vi "Actor Core.vi"(8 "error in":errorcluster, 11 "Multiharp in":refnum<class "Multiharp.lvclass">) -> (0 "error out":errorcluster, 3 "Actor out":refnum<class "Actor.lvclass">)   [LabVIEW 2023, in "Multiharp.lvlib" / "Multiharp.lvclass"]
doc: "(<B>Filename</B>: Actor Framework.lvlib:Actor.lvclass:Actor Core.vi)\n\nReceives messages to the actor, reacts to them, and initiates any error handling that may shut the actor down.\n\nDescendant classes may override this VI to append parallel tasks for the actor to complete while it handles messages. Overrides use the Call Parent Class Method node."
uses:
  Multiharp.lvclass
  C:/Program Files/National Instruments/LabVIEW 2023/vi.lib/ActorFramework/Actor/Actor.lvclass
  <vilib>/ActorFramework/Actor/Actor.lvclass
  MH_ActorCluster.ctl
  Types/MH_DataProcThread_QData.ctl
  Types/MH_DataProcThread_QCmds.ctl
  UIs/SinglePhoton_UI/Libraries/SinglePhotonInterferenceUI/CountsHistos.ctl
  <vilib>/ActorFramework/Message Enqueuer/Message Enqueuer.lvclass
  <vilib>/ActorFramework/Actor/Actor.lvclass/Actor.ctl
  <vilib>/ActorFramework/Message Enqueuer/Message Enqueuer.lvclass/Message Enqueuer.ctl
  Multiharp.lvclass/Multiharp.ctl
  MultiharpComm Messages/MH_MeasurementDone Msg/MH_MeasurementDone Msg.lvclass/MH_MeasurementDone Msg.ctl
  MultiharpComm Messages/MH_DataInQueue Msg/MH_DataInQueue Msg.lvclass/MH_DataInQueue Msg.ctl
  <vilib>/ActorFramework/Message Enqueuer/Init from Existing Queue.vi
  <vilib>/ActorFramework/Message Enqueuer/Enqueue.vi
  Multiharp Messages/StopMeasurement Msg/StopMeasurement Msg.lvclass
  C:/Program Files/National Instruments/LabVIEW 2023/vi.lib/ActorFramework/Message/Message.lvclass
  MultiharpComm Messages/MH_MeasurementDone Msg/MH_MeasurementDone Msg.lvclass
  MultiharpComm Messages/MH_DataInQueue Msg/MH_DataInQueue Msg.lvclass
  <vilib>/ActorFramework/Message Priority Queue/Priority Enqueue.vi
  typedefs/typedefs.lvlib
panel:
  out "UI Enqueuer":refnum<class "Message Enqueuer.lvclass">
  out "Self Enqueuer":refnum<class "Message Enqueuer.lvclass">
  in  "CountsHistos":T1
  in  "CountsHistos":T1
  in  "FIFO Buffer":T2={"Cmd"=enum."Proc", "nActual"=0, "Buffer"=[], "TickCount"=0, "Param"=0, "Max Triggers"=0, "Coincidence Window"=2.0, "Coincidence Delays"=[], "file path"=path ""}
  in  "MH_ActorCluster":T4={"Histo On"=FALSE, "Initialized"=FALSE, "Acquiring"=FALSE, "ActualHistoLe"=0, "Scanning"=TRUE, "nchannels"=0, "file path"=path "", "BufferSize"=[]}
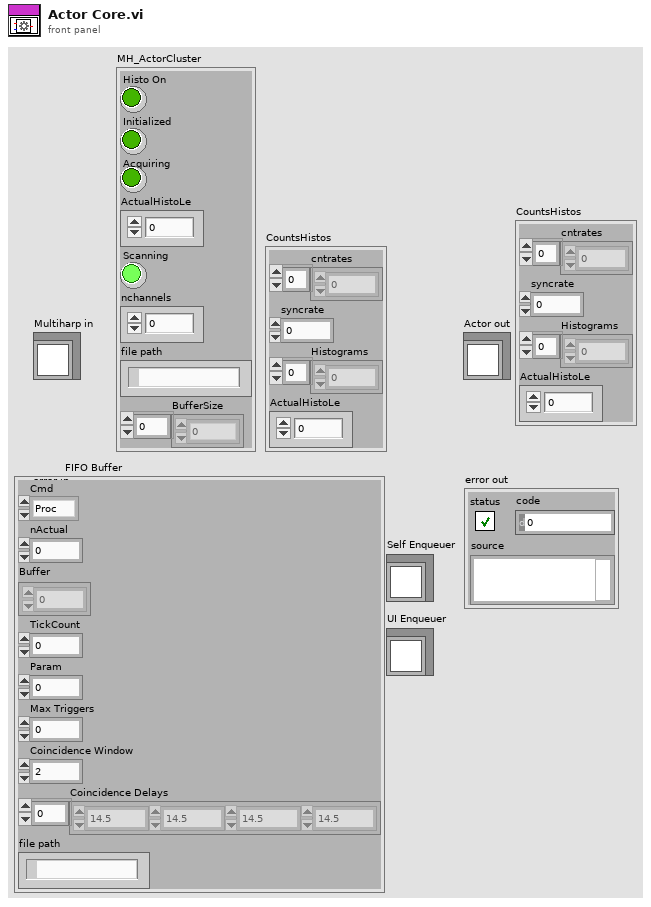
[diagram p1: front panel]
types:
  T1 = typedef "typedefs.lvlib/CountsHistos.ctl" = cluster{"cntrates":i32[], "syncrate":i32, "Histograms":u32[], "ActualHistoLe":i32}
  T2 = typedef "MH_DataProcThread_QData.ctl" = cluster{"Cmd":T3, "nActual":i32, "Buffer":u32[], "TickCount":u32, "Param":i32, "Max Triggers":i32, "Coincidence Window":dbl, "Coincidence Delays":dbl[], "file path":path}
  T3 = typedef "MH_DataProcThread_QCmds.ctl" = enum16{"Exit", "Proc", "Init", "SaveCSV", "SetNumChannels"}
  T4 = typedef "MH_ActorCluster.ctl" = cluster{"Histo On":bool, "Initialized":bool, "Acquiring":bool, "ActualHistoLe":i32, "Scanning":bool, "nchannels":i32, "file path":path, "BufferSize":dbl[]}
  T5 = enum16{"Idle", "Scanning", "Acquiring", "Histogramming", "Counting"}
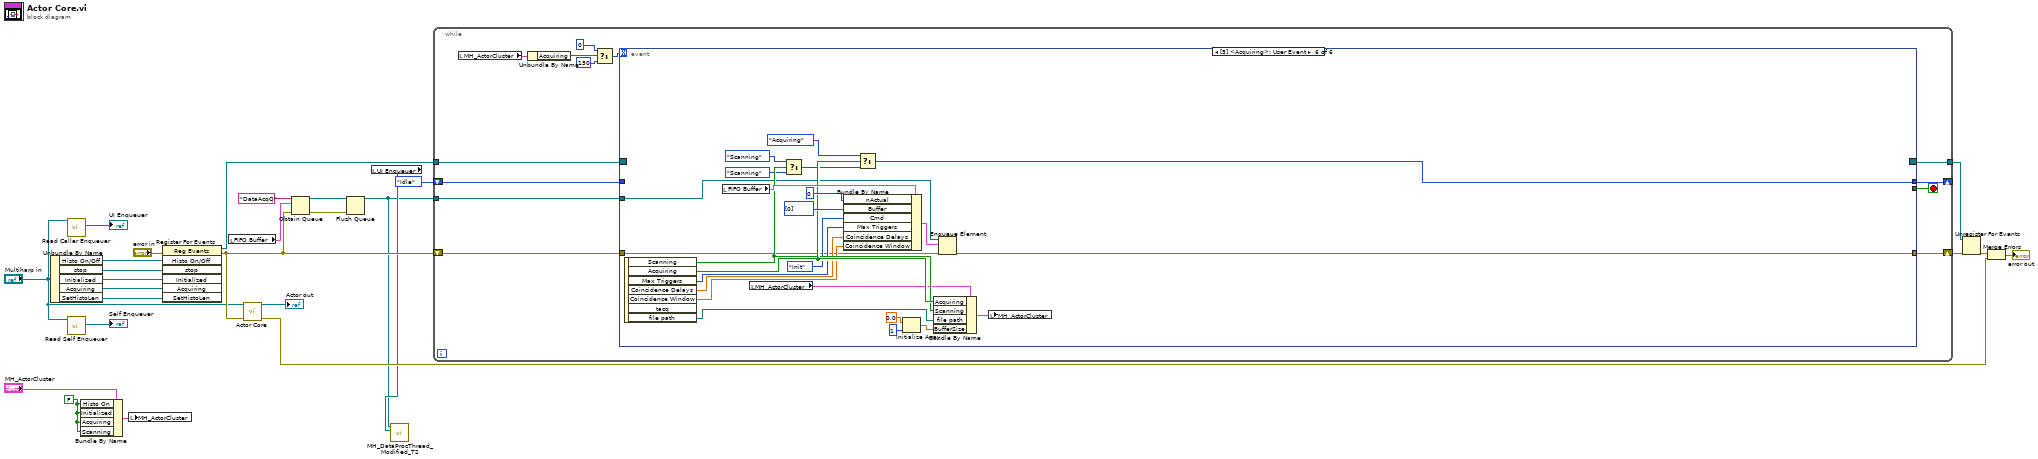
[diagram p0: block diagram]
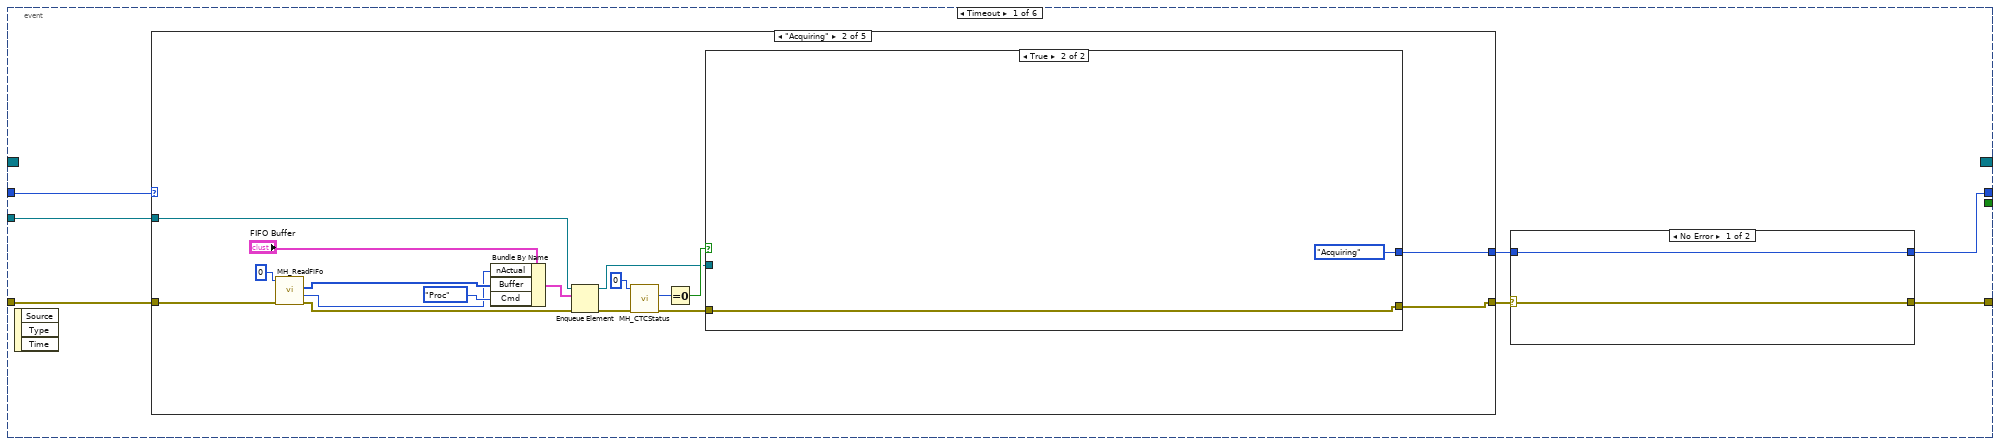
[diagram p2: hidden frame]
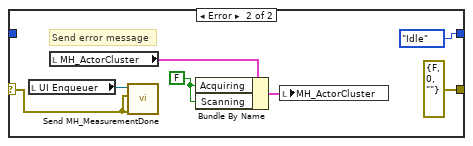
[diagram p3: hidden frame]
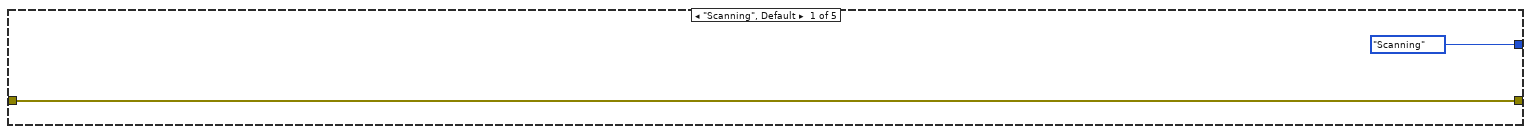
[diagram p4: hidden frame]
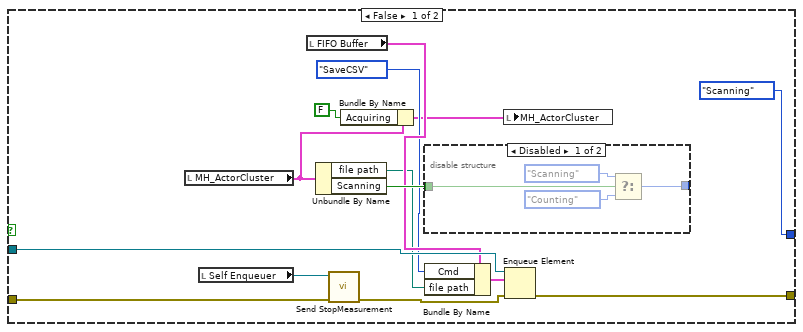
[diagram p5: hidden frame]
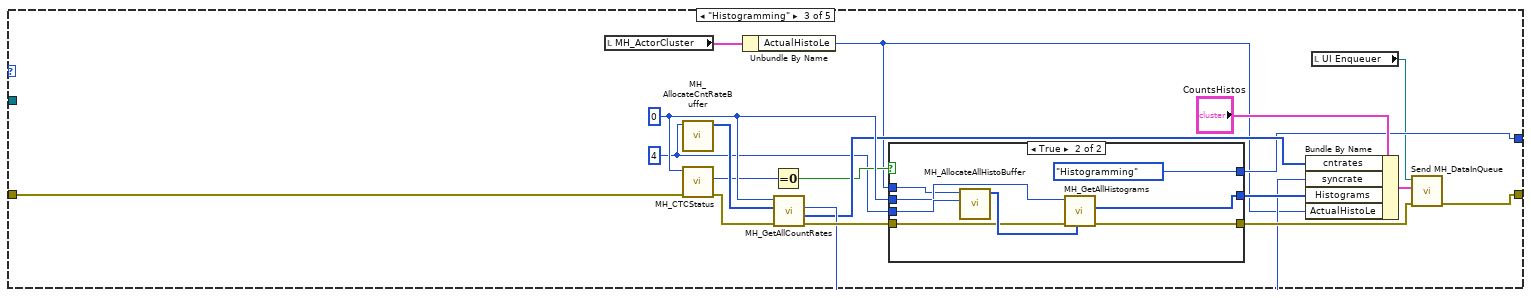
[diagram p7: hidden frame]
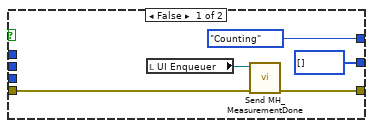
[diagram p8: hidden frame]
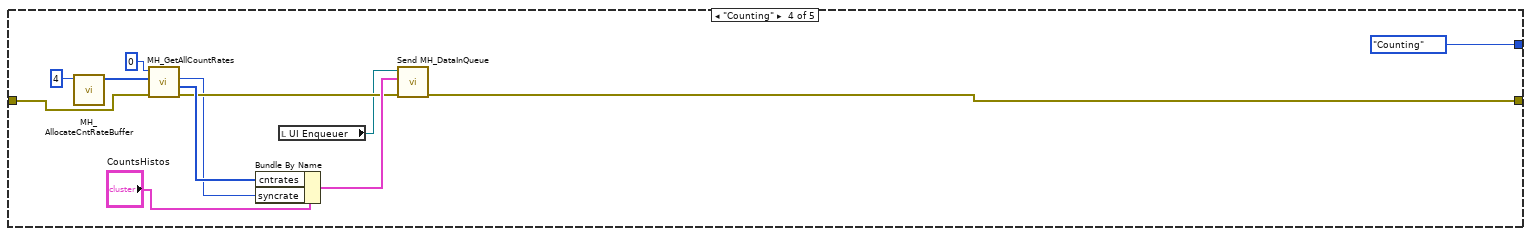
[diagram p9: hidden frame]
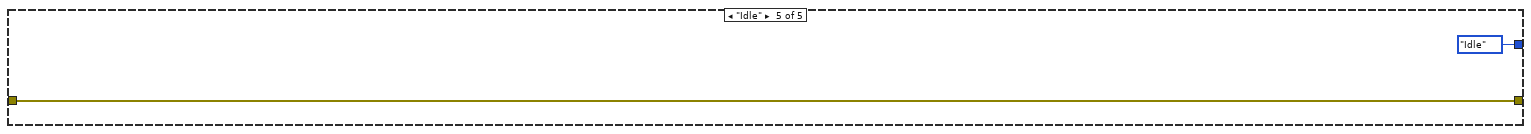
[diagram p10: hidden frame]
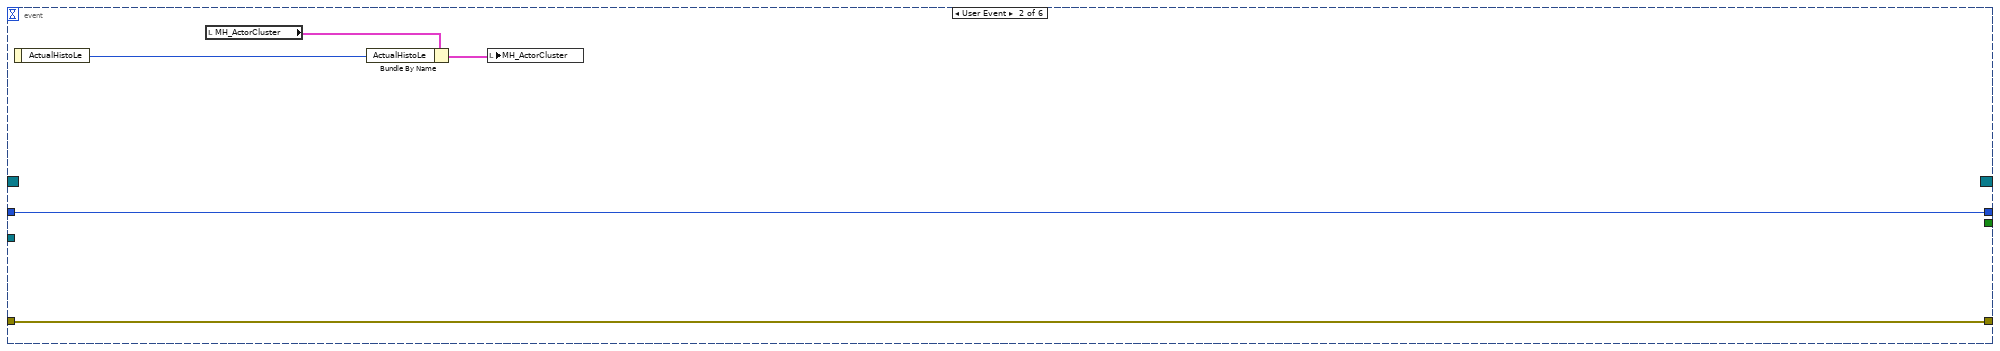
[diagram p11: hidden frame]
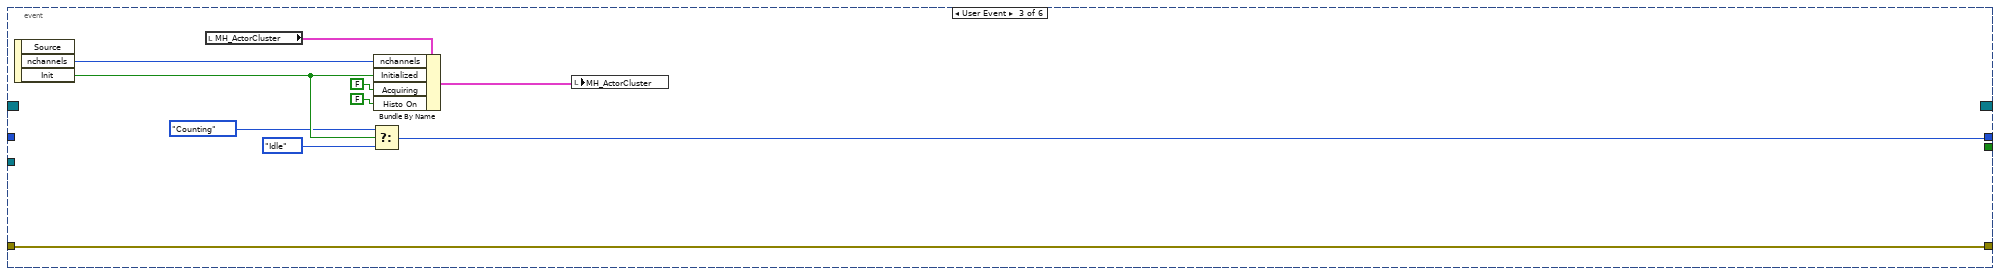
[diagram p12: hidden frame]
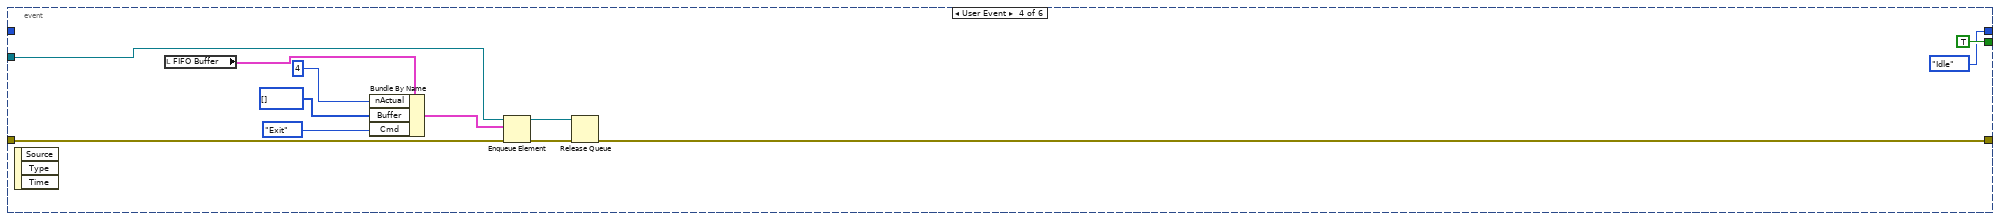
[diagram p13: hidden frame]
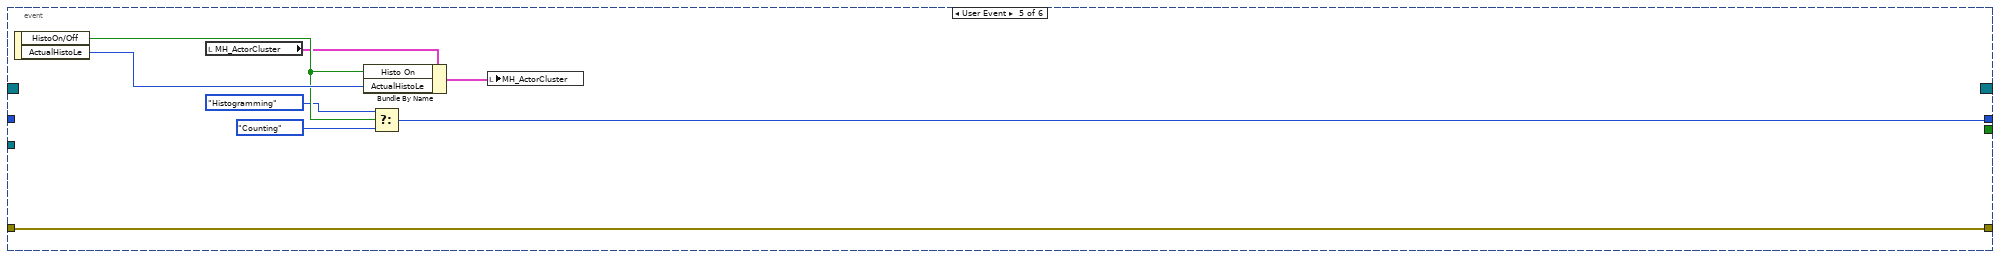
[diagram p14: hidden frame]
diagram:
  w14 = FALSE ("Histo On")
  n1 = Unbundle By Name("Multiharp in") -> ("Histo On/Off"=w25:refnum<user-event>, "stop"=w23:refnum<user-event>, "Initialized"=w22:refnum<user-event>, "Acquiring"=w18:refnum<user-event>, "SetHistoLen"=w15:refnum<user-event>)
  n2 = call <vilib>:"Read Caller Enqueuer.vi"("Actor"="Multiharp in") -> ("Caller Enqueuer"=→"UI Enqueuer":refnum<class "Message Enqueuer.lvclass">)  [unwired: 10 in]
  n3 = call <vilib>:"Read Self Enqueuer.vi"("Actor"="Multiharp in") -> ("Self Enqueuer"=→"Self Enqueuer":refnum<class "Message Enqueuer.lvclass">)  [unwired: 10 in]
  n4 = Bundle By Name(cluster="MH_ActorCluster", "Histo On"=w14, "Initialized"=w14, "Acquiring"=w14, "Scanning"=w14) -> (w4:T4)
  n5 = local write "MH_ActorCluster"(w4) -> ()
  n6 = register-events(error in="error in", w25, w23, w22, w18, w15) -> (reference out=w26:refnum<event-registration>, error out=w8:errorcluster)  [unwired: 1 in]
  n7 = local read "FIFO Buffer"() -> (w17:T2)
  n8 = call-parent "Actor Core.vi"("error in"=w8, "Actor in"="Multiharp in") -> ("error out"=w21:errorcluster, "Actor out"=→"Actor out":refnum<class "Actor.lvclass">)  [unwired: 8 in]
  n9 = Obtain Queue(name (unnamed)="DataAcqQ", element data type=w17, error in (no error)=w8) -> (queue out=w1:refnum<queue>, error out=w2:errorcluster)  [unwired: 2 in, 1 out]
  n10 = Flush Queue(queue=w1, error in (no error)=w2) -> (queue out=w3:refnum<queue>)  [unwired: 2 out]
  n11 = local read "UI Enqueuer"() -> (w5:refnum<class "Message Enqueuer.lvclass">)
  n12 = call "MH_DataProcThread_Modified_T2.vi"("Message Enqueuer"=w5, "MH_DataProcThread_QRef"=w3) -> ()  [unwired: 10 in]
  n13 = while {
    shift-right: [w40] -> w10
    shift-left: w8 -> [w39]
    tunnel: w26 -> [w38]
    tunnel: [w37] -> w24
    tunnel: w3 -> [w35]
    shift-right: [w33] -> _
    shift-left: T5."Idle" -> [w34]
    stop <- w36 stop-if-true
    n14 = local read "MH_ActorCluster"() -> (w29:T4)
    n15 = Unbundle By Name(w29) -> ("Acquiring"=w28:bool)
    n16 = Select(t=0, s=w28, f=150) -> (s? t:f=w30:i32)
    n17 = event shown="[5] <Acquiring>: User Event" {
      selector: w38 -> [_ _ _ _ _ _]
      dyn-events: [_ _ _ _ _ _] -> w37
      timeout: w30 -> [_ _ _ _ _ _]
      tunnel: [w47 w145 w156 w158 w171 w177] -> w40
      tunnel: w39 -> [w46 w145 w156 w159 w171 w178]
      tunnel: [_ _ _ TRUE _ _] -> w36
      tunnel: w35 -> [w45 _ _ w161 _ w184]
      tunnel: w34 -> [w42 w144 _ _ _ _]
      tunnel: [w43 w144 w149 T5."Idle" w172 w190] -> w33
      event Timeout {
        n18 = event-data() -> ()  [unwired: 1 in, 3 out]
        n19 = case shown="\"Acquiring\"" w42 {
          tunnel: [w58 w69 w103 w137 w141] -> w41
          tunnel: w46 -> [w58 w59 w102 w136 w141]
          tunnel: w45 -> [_ w67 _ _ _]
          tunnel: [T5."Scanning" ("f") w73 w100 T5."Counting" ("f") T5."Idle" ("f")] -> w44
          frame "Scanning", Default {
          }
          frame "Acquiring" {
            n20 = call "MH_ReadFiFo.vi"("error in (no error)"=w59, "devidx"=0) -> ("error out"=w68:errorcluster, "nactual"=w65:i32, "buffer"=w66:u32[])  [unwired: 6 in, 1 out]
            n21 = Bundle By Name(cluster="FIFO Buffer", "nActual"=w65, "Buffer"=w66, "Cmd"=MH_DataProcThread_QCmds."Proc") -> (w72:T2)
            n22 = Enqueue Element(queue=w67, element=w72, error in (no error)=w68) -> (queue out=w64:refnum<queue>, error out=w62:errorcluster)  [unwired: 1 in, 1 out]
            n23 = call "MH_CTCStatus.vi"("error in (no error)"=w62, "devidx"=0) -> ("error out"=w61:errorcluster, "ctcstatus"=w60:i32)  [unwired: 7 in, 1 out]
            n24 = Equal To 0?(x=w60) -> (x = 0?=w75:bool)
            n25 = case shown="True" w75 {
              tunnel: [w82 w94] -> w69
              tunnel: w61 -> [w81 w94]
              tunnel: w64 -> [w86 _]
              tunnel: [T5."Scanning" ("f") T5."Acquiring"] -> w73
              frame False {
                n26 = local read "MH_ActorCluster"() -> (w77:T4)
                n27 = local read "Self Enqueuer"() -> (w78:refnum<class "Message Enqueuer.lvclass">)
                n28 = local read "FIFO Buffer"() -> (w85:T2)
                n29 = Unbundle By Name(w77) -> ("file path"=w83:path, "Scanning"=w88:bool)
                n30 = call "Send StopMeasurement.vi"("error in (no error)"=w81, "Message Enqueuer"=w78) -> ("error out"=w80:errorcluster)  [unwired: 8 in, 1 out]
                n31 = Bundle By Name(cluster=w77, "Acquiring"=FALSE) -> (w76:T4)
                n32 = disable-structure shown="Disabled" {
                  disable-tunnel: w88 -> [w93 _]
                  disable-tunnel: [w92 _] -> _
                  frame Disabled {
                    n33 = Select(t=T5."Scanning", s=w93, f=T5."Counting") -> (s? t:f=w92:T5)
                  }
                  frame Enabled {
                  }
                }
                n34 = Bundle By Name(cluster=w85, "Cmd"=MH_DataProcThread_QCmds."SaveCSV", "file path"=w83) -> (w87:T2)
                n35 = local write "MH_ActorCluster"(w76) -> ()
                n36 = Enqueue Element(queue=w86, element=w87, error in (no error)=w80) -> (error out=w82:errorcluster)  [unwired: 1 in, 2 out]
              }
              frame True {
              }
            }
          }
          frame "Histogramming" {
            w99 = 4 ("NumChan")
            w112 = 0 ("devidx")
            n37 = local read "MH_ActorCluster"() -> (w96:T4)
            n38 = call "MH_AllocateCntRateBuffer.vi"("NumChan"=w99) -> ("Buffer"=w106:i32[])  [unwired: 10 in]
            n39 = call "MH_CTCStatus.vi"("error in (no error)"=w102, "devidx"=w112) -> ("error out"=w101:errorcluster, "ctcstatus"=w105:i32)  [unwired: 7 in, 1 out]
            n40 = Unbundle By Name(w96) -> ("ActualHistoLe"=w98:i32)
            n41 = Equal To 0?(x=w105) -> (x = 0?=w104:bool)
            n42 = call "MH_GetAllCountRates.vi"("error in (no error)"=w101, "cntrates_buf"=w106, "devidx"=w112) -> ("error out"=w113:errorcluster, "cntrates"=w109:i32[], "syncrate"=w110:i32)  [unwired: 5 in, 1 out]
            n43 = case shown="True" w104 {
              tunnel: w99 -> [_ w126]
              tunnel: [u32[] [] ("Histograms") w125] -> w111
              tunnel: w113 -> [w118 w124]
              tunnel: [w117 w123] -> w114
              tunnel: w112 -> [_ w122]
              tunnel: [T5."Counting" ("f") T5."Histogramming" ("f")] -> w100
              tunnel: w98 -> [_ w120]
              frame False {
                n44 = local read "UI Enqueuer"() -> (w115:refnum<class "Message Enqueuer.lvclass">)
                n45 = call "Send MH_MeasurementDone.vi"("error in (no error)"=w118, "Message Enqueuer"=w115) -> ("error out"=w117:errorcluster)  [unwired: 8 in, 1 out]
              }
              frame True {
                n46 = call "MH_AllocateAllHistoBuffer.vi"("NumChan"=w126, "HistoLength"=w120) -> ("Buffer"=w127:u32[])  [unwired: 9 in]
                n47 = call "MH_GetAllHistograms.vi"("Chcount"=w127, "error in (no error)"=w124, "devidx"=w122) -> ("error out"=w123:errorcluster, "Histograms"=w125:u32[])  [unwired: 6 in, 1 out]
              }
            }
            n48 = Bundle By Name(cluster="CountsHistos", "cntrates"=w109, "syncrate"=w110, "Histograms"=w111, "ActualHistoLe"=w98) -> (w107:T1)
            n49 = local read "UI Enqueuer"() -> (w97:refnum<class "Message Enqueuer.lvclass">)
            n50 = call "Send MH_DataInQueue.vi"("error in (no error)"=w114, "CountsHistos"=w107, "Message Enqueuer"=w97) -> ("error out"=w103:errorcluster)  [unwired: 7 in, 1 out]
          }
          frame "Counting" {
            n51 = call "MH_AllocateCntRateBuffer.vi"("NumChan"=4) -> ("Buffer"=w139:i32[])  [unwired: 10 in]
            n52 = call "MH_GetAllCountRates.vi"("error in (no error)"=w136, "cntrates_buf"=w139, "devidx"=0) -> ("error out"=w131:errorcluster, "cntrates"=w134:i32[], "syncrate"=w129:i32)  [unwired: 5 in, 1 out]
            n53 = Bundle By Name(cluster="CountsHistos", "cntrates"=w134, "syncrate"=w129) -> (w132:T1)
            n54 = local read "UI Enqueuer"() -> (w128:refnum<class "Message Enqueuer.lvclass">)
            n55 = call "Send MH_DataInQueue.vi"("error in (no error)"=w131, "CountsHistos"=w132, "Message Enqueuer"=w128) -> ("error out"=w137:errorcluster)  [unwired: 7 in, 1 out]
          }
          frame "Idle" {
          }
        }
        n56 = case shown="No Error" w41 {
          selector: w41 -> [w49 w55]
          tunnel: [w49 errorcluster {"status"=FALSE, "code"=0, "source"=""} ("error IO")] -> w47
          tunnel: w44 -> [w48 _]
          tunnel: [w48 T5."Idle" ("f")] -> w43
          frame No Error {
          }
          frame Error {
            w54 = FALSE ("Acquiring")
            # "Send error message"
            n57 = local read "UI Enqueuer"() -> (w52:refnum<class "Message Enqueuer.lvclass">)
            n58 = local read "MH_ActorCluster"() -> (w51:T4)
            n59 = call "Send MH_MeasurementDone.vi"("error in (no error)"=w55, "MH_Meas_Error"=w55, "Message Enqueuer"=w52) -> ()  [unwired: 7 in, 2 out]
            n60 = Bundle By Name(cluster=w51, "Acquiring"=w54, "Scanning"=w54) -> (w50:T4)
            n61 = local write "MH_ActorCluster"(w50) -> ()
          }
        }
      }
      event User Event {
        n62 = event-data() -> ("ActualHistoLe"=w146:i32)  [unwired: 1 in]
        n63 = local read "MH_ActorCluster"() -> (w142:T4)
        n64 = Bundle By Name(cluster=w142, "ActualHistoLe"=w146) -> (w143:T4)
        n65 = local write "MH_ActorCluster"(w143) -> ()
      }
      event User Event {
        n66 = event-data() -> ("nchannels"=w153:i32, "Init"=w152:bool)  [unwired: 1 in, 1 out]
        n67 = local read "MH_ActorCluster"() -> (w148:T4)
        n68 = Select(t=T5."Counting", s=w152, f=T5."Idle") -> (s? t:f=w149:T5)
        n69 = Bundle By Name(cluster=w148, "nchannels"=w153, "Initialized"=w152, "Acquiring"=FALSE, "Histo On"=FALSE) -> (w147:T4)
        n70 = local write "MH_ActorCluster"(w147) -> ()
      }
      event User Event {
        n71 = event-data() -> ()  [unwired: 1 in, 3 out]
        n72 = local read "FIFO Buffer"() -> (w163:T2)
        n73 = Bundle By Name(cluster=w163, "nActual"=4, "Buffer"=u32[] [], "Cmd"=MH_DataProcThread_QCmds."Exit") -> (w165:T2)
        n74 = Enqueue Element(queue=w161, element=w165, error in (no error)=w159) -> (queue out=w157:refnum<queue>, error out=w160:errorcluster)  [unwired: 1 in, 1 out]
        n75 = Release Queue(queue=w157, error in (no error)=w160) -> (error out=w158:errorcluster)  [unwired: 1 in, 2 out]
      }
      event User Event {
        n76 = event-data() -> ("HistoOn/Off"=w175:bool, "ActualHistoLe"=w176:i32)  [unwired: 1 in]
        n77 = local read "MH_ActorCluster"() -> (w170:T4)
        n78 = Bundle By Name(cluster=w170, "Histo On"=w175, "ActualHistoLe"=w176) -> (w169:T4)
        n79 = Select(t=T5."Histogramming", s=w175, f=T5."Counting") -> (s? t:f=w172:T5)
        n80 = local write "MH_ActorCluster"(w169) -> ()
      }
      event User Event {
        n81 = event-data() -> ("Scanning"=w194:bool, "Acquiring"=w196:bool, "Max Triggers"=w189:i32, "Coincidence Delays"=w187:dbl[], "Coincidence Window"=w186:dbl, "file path"=w185:path)  [unwired: 1 in, 1 out]
        n82 = local read "FIFO Buffer"() -> (w198:T2)
        n83 = local read "MH_ActorCluster"() -> (w180:T4)
        n84 = Select(t=T5."Scanning", s=w194, f=T5."Scanning") -> (s? t:f=w191:T5)
        n85 = Bundle By Name(cluster=w198, "nActual"=0, "Buffer"=u32[] [0], "Cmd"=MH_DataProcThread_QCmds."Init", "Max Triggers"=w189, "Coincidence Delays"=w187, "Coincidence Window"=w186) -> (w197:T2)
        n86 = Select(t=T5."Acquiring", s=w196, f=w191) -> (s? t:f=w190:T5)
        n87 = Initialize Array(0.0 ("element"), 1 ("dimension size")) -> (w183:dbl[])
        n88 = Bundle By Name(cluster=w180, "Acquiring"=w196, "Scanning"=w194, "file path"=w185, "BufferSize"=w183) -> (w179:T4)
        n89 = Enqueue Element(queue=w184, element=w197, error in (no error)=w178) -> (error out=w177:errorcluster)  [unwired: 1 in, 2 out]
        n90 = local write "MH_ActorCluster"(w179) -> ()
      }
    }
  }
  n91 = Unregister For Events(event registration refnum=w24, error in=w10) -> (error out=w9:errorcluster)
  n92 = Merge Errors(w9, w21) -> (→"error out":errorcluster)
